vi "Nodes.vi"(8 "error in (no error)":errorcluster, 11 "Cluster in":refnum<class "Cluster.lvclass">) -> (0 "error out":errorcluster, 2 "Nodes":refnum<class "Node.lvclass">[](array[class]), 3 "Cluster out":refnum<class "Cluster.lvclass">)   [LabVIEW 2020, in "VolatusConfig.lvlib" / "Cluster.lvclass"]
uses:
  Cluster.lvclass
  Cluster.lvclass/Cluster.ctl
  VolatusConfigElement/VolatusConfigElement.lvclass
  VolatusConfig.lvlib
  Meta Type.ctl
  Node/Node.lvclass
  C:/dev/lv20CE/relink/lv-volatus/VolatusConfig/VolatusConfigElement/VolatusConfigElement.lvclass
  C:/dev/lv20CE/relink/lv-volatus/VolatusConfig/Cluster/Cluster.lvclass
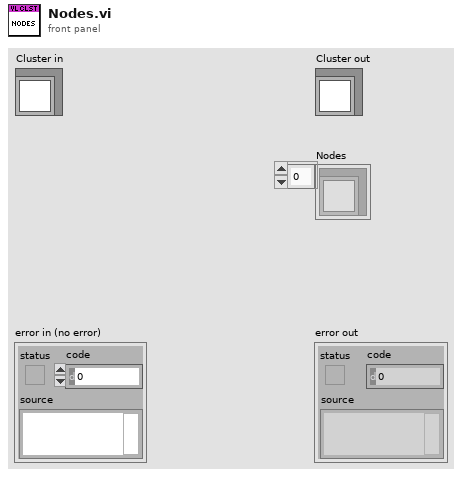
[diagram p1: front panel]
types:
  T1 = typedef "VolatusConfig.lvlib/Meta Type.ctl" = enum16{"UNKNOWN", "VL_System", "VL_Cluster", "VL_Node", "VL_Task", "VL_Group", "VL_Channel", "VL_Task_List", "VL_Scaling", "VL_Sensor", "VL_Sensor_List", "VL_Scale"}
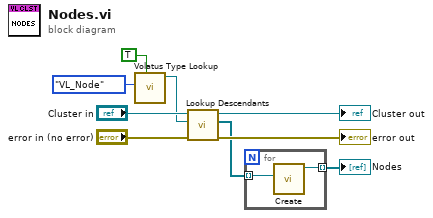
[diagram p0: block diagram]
diagram:
  n1 = call "Volatus Type Lookup.vi"("Don't Recurse Past Match (F)"=TRUE, "Meta Type"=Meta_Type."VL_Node") -> ("Config Lookup out"=w3:refnum<class "Config Lookup.lvclass">)  [unwired: 8 in, 1 out]
  n2 = call "Lookup Descendants.vi"("error in (no error)"="error in (no error)", "Lookup"=w3, "VolatusConfigElement in"="Cluster in") -> ("error out"=→"error out":errorcluster, "Descendants"=w2:refnum<class "Config Element.lvclass">[], "VolatusConfigElement out"=→"Cluster out":refnum<class "Cluster.lvclass">)  [unwired: 6 in]
  n3 = for {
    tunnel: w2 -> [w11] mode=indexing
    tunnel: [w10] -> w1 mode=indexing
    n4 = call "Create.vi"("Element"=w11) -> ("Node out"=w10:refnum<class "Node.lvclass">)  [unwired: 9 in, 1 out]
  }
  "Nodes" <- w1
